vi "Update Assert Failure Action.vi"(8 "error in (no error)":errorcluster, 9 "Assert Name":string, 10 "Target Failure Action":string, 11 "AssertEngine in":refnum<class "AssertEngine.lvclass">) -> (0 "error out":errorcluster, 3 "AssertEngine out":refnum<class "AssertEngine.lvclass">)   [LabVIEW 2016, in "AssertEngine.lvlib" / "AssertEngine.lvclass"]
uses:
  AssertEngine.lvclass
  Log Assert/Assert Data.ctl
  AssertEngine.lvclass/AssertEngine.ctl
  AssertEngine.lvlib
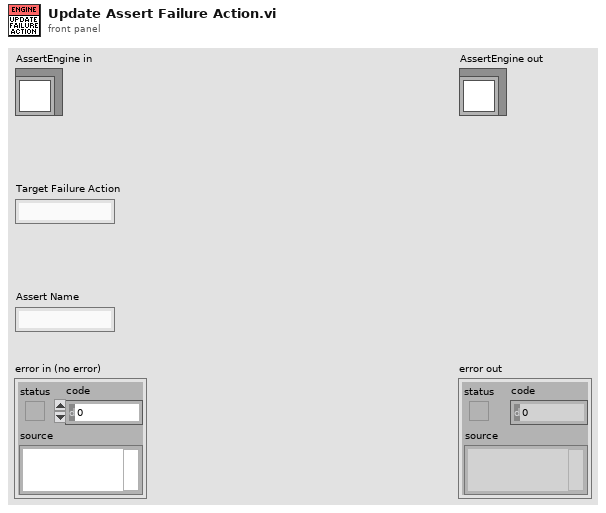
[diagram p1: front panel]
types:
  T1 = typedef "AssertEngine.lvlib/Assert Data.ctl" = cluster{"Assert Name":string, "Status":string, "Comment":string, "Eval String":string, "Failure Action":string, "Calling VI Name":string, "Assert VI Name":string, "Data Value":variant, "Assert VI UID":i32, "Assert Builder":string, "Build Timestamp":timestamp, "Last Update (Date)":string, "Top Level VI Name":string, "Data Type":string, "Last Update (Time)":string}
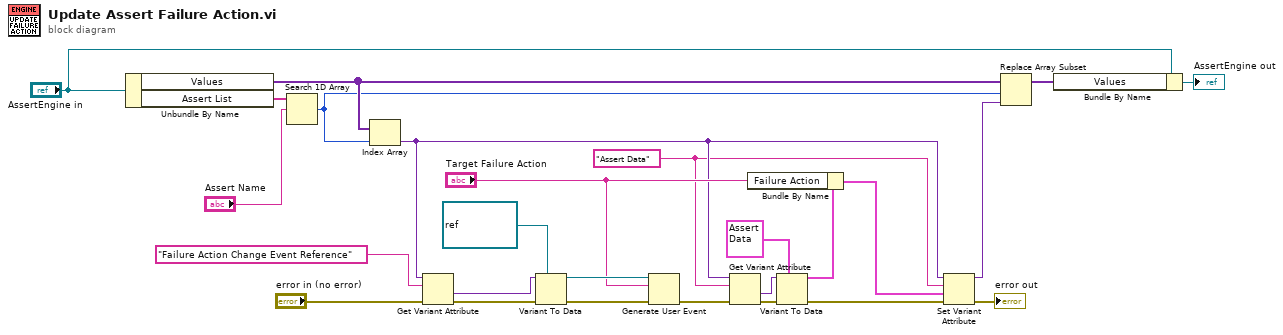
[diagram p0: block diagram]
diagram:
  w7 = "Assert Data"
  n1 = Unbundle By Name("AssertEngine in") -> ("Values"=w5:variant[], "Assert List"=w24:string[])
  n2 = Search 1D Array(1D array=w24, element="Assert Name") -> (index of element=w3:i32)  [unwired: 1 in]
  n3 = Index Array(array=w5, index=w3) -> (element=w8:variant)
  n4 = Get Variant Attribute(Variant=w8, name="Failure Action Change Event Reference", error in="error in (no error)") -> (value=w19:variant, error out=w22:errorcluster)  [unwired: 1 in, 2 out]
  n5 = Variant To Data(error in=w22, type=refnum<user-event> refnum ("Failure Action Change Event"), Variant=w19) -> (data=w16:refnum<user-event>, error out=w20:errorcluster)
  n6 = Generate User Event(user event=w16, event data cluster="Target Failure Action", error in=w20) -> (error out=w17:errorcluster)  [unwired: 1 in, 1 out]
  n7 = Get Variant Attribute(Variant=w8, name=w7, error in=w17) -> (value=w13:variant, error out=w15:errorcluster)  [unwired: 1 in, 2 out]
  n8 = Variant To Data(error in=w15, type=T1 {"Assert Name"="", "Status"="", "Comment"="", "Eval String"="", "Failure Action"="", "Calling VI Name"="", "Assert VI Name"="", "Data Value"=variant, "Assert VI UID"=0, "Assert Builder"="", "Build Timestamp"=timestamp(0 s since 1904-01-01), "Last Update (Date)"="", "Top Level VI Name"="", "Data Type"="", "Last Update (Time)"=""} ("Assert Data"), Variant=w13) -> (data=w11:T1, error out=w14:errorcluster)
  n9 = Bundle By Name(cluster=w11, "Failure Action"="Target Failure Action") -> (w6:T1)
  n10 = Set Variant Attribute(Variant=w8, name=w7, value=w6, error in=w14) -> (Variant out=w4:variant, error out=→"error out":errorcluster)  [unwired: 1 out]
  n11 = Replace Array Subset(array=w5, new element=w4, index=w3) -> (w1:variant[])
  n12 = Bundle By Name(cluster="AssertEngine in", "Values"=w1) -> (→"AssertEngine out":refnum<class "AssertEngine.lvclass">)
